vi "Initiate Acquisition.vi"(8 "error in (no error)":errorcluster {"code" format="%.0x"}, 11 "VISA Resource Name":refnum<visa-resource-name>) -> (0 "error out":errorcluster {"code" format="%.0x"}, 3 "VISA Resource Name Out":refnum<visa-resource-name>)   [LabVIEW 2010, in "Tektronix TDS 3000 Series.lvlib"]
doc: "This VI initiates a waveform acquisition. After you call this VI, the oscilloscope leaves the Idle state and waits for a trigger. The oscilloscope acquires a waveform for each channel you have enabled with the tktds3k Configure Channel VI.\n\nNotes:\n\n(1) Typically, you call this VI only in a sequence of calls to other low-level driver VIs. The sequence performs one operation. You use the low-level VIs to optimize one or more aspects of interaction with the instrument. If you want to check the instrument status, call the tktds3k Error-Query VI at the conclusion of the sequence."
uses:
  <instrlib>/Tektronix TDS 3000 Series/Tektronix TDS 3000 Series.lvlib
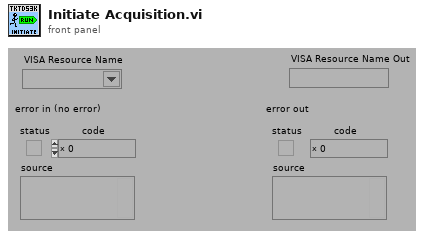
[diagram p1: front panel]
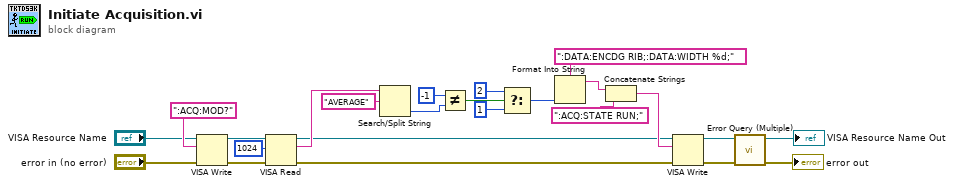
[diagram p0: block diagram]
diagram:
  n1 = VISA Write(VISA resource name="VISA Resource Name", write buffer=":ACQ:MOD?", error in (no error)="error in (no error)") -> (VISA resource name out=w22:refnum<visa-resource-name>, error out=w23:errorcluster)  [unwired: 1 out]
  n2 = VISA Read(VISA resource name=w22, byte count=1024, error in (no error)=w23) -> (VISA resource name out=w5:refnum<visa-resource-name>, read buffer=w14:string, error out=w6:errorcluster)  [unwired: 1 out]
  n3 = Search/Split String(string=w14, search string/char (-)="AVERAGE") -> (offset of match=w12:i32)  [unwired: 1 in, 2 out]
  n4 = Not Equal?(x=-1, y=w12) -> (x != y?=w13:bool)
  n5 = Select(t=u32 2, s=w13, f=u32 1) -> (s? t:f=w7:u32)
  n6 = Format Into String(format string=":DATA:ENCDG RIB;:DATA:WIDTH %d;", w7) -> (resulting string=w9:string)  [unwired: 2 in, 1 out]
  n7 = Concatenate Strings(w9, ":ACQ:STATE RUN;" ("string")) -> (w8:string)
  n8 = VISA Write(VISA resource name=w5, write buffer=w8, error in (no error)=w6) -> (VISA resource name out=w4:refnum<visa-resource-name>, error out=w3:errorcluster)  [unwired: 1 out]
  n9 = call <instrlib>:"Error Query (Multiple).vi"("error in (no error)"=w3, "VISA Resource Name"=w4) -> ("error out"=→"error out":errorcluster, "VISA Resource Name Out"=→"VISA Resource Name Out":refnum<visa-resource-name>)  [unwired: 6 in, 2 out]
